vi "Set Column Widths.vi"(8 "error in (no error)":errorcluster, 10 "Column Widths":u32[](array[numeric]), 11 "AppMgr in":refnum<class "Application Manager.lvclass">) -> (0 "error out":errorcluster, 3 "AppMgr out":refnum<class "Application Manager.lvclass">)   [LabVIEW 2017, in "Application Manager.lvclass"]
uses:
  Application Manager.lvclass
  Application Manager.lvclass/Application Manager.ctl
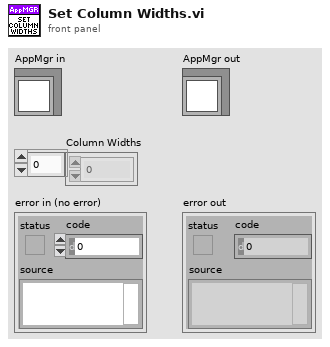
[diagram p1: front panel]
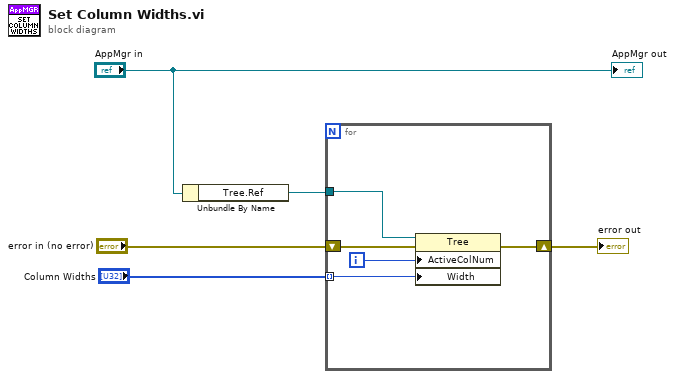
[diagram p0: block diagram]
diagram:
  n1 = Unbundle By Name("AppMgr in") -> ("Tree.Ref"=w4:refnum<vi>)
  n2 = for {
    tunnel: w4 -> [w10]
    shift-right: [w8] -> w1
    shift-left: "error in (no error)" -> [w9]
    tunnel: "Column Widths" -> [w6] mode=indexing
    i -> [w7]
    n3 = property class="Tree"(reference=w10, error in=w9, "ActiveColNum"=w7, "Width"=w6) -> (error out=w8:errorcluster)  [unwired: 1 out]
  }
  "error out" <- w1
  "AppMgr out" <- "AppMgr in"
